vi "Get Connection to Detector.vi"(6 "BAUD":u16, 7 "Mode":enum16{"RTU", "ASCII"}(ring), 8 "error in (no error)":errorcluster, 9 "Порт":u16, 10 "find list":string[](array[string]), 11 "Адрес датчика":u16) -> (0 "error out":errorcluster, 1 "SN":u16, 2 "FW":u16, 3 "VISA Refnum out":refnum<visa-resource-name>, 4 "p_atm":sgl, 5 "Cluster":T1)   [LabVIEW 2020]
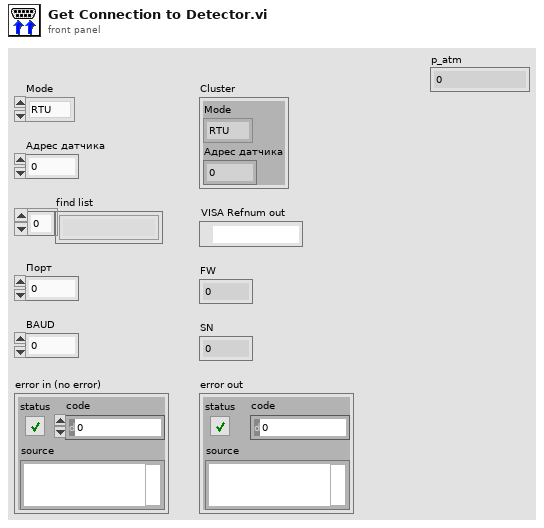
[diagram p1: front panel]
types:
  T1 = cluster{"Mode":enum16{"RTU", "ASCII"}, "Адрес датчика":u16}
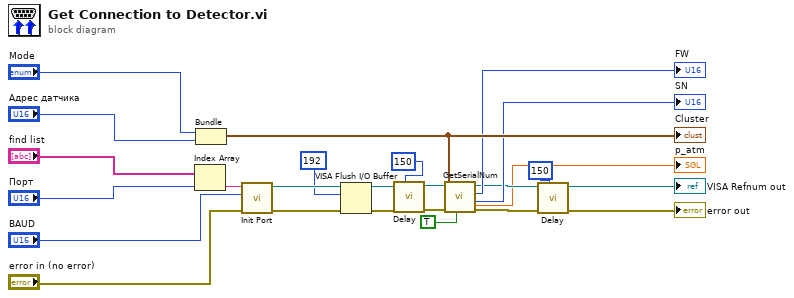
[diagram p0: block diagram]
diagram:
  n1 = Index Array(array="find list", index="Порт") -> (element=w12:string)
  n2 = Bundle("Mode"="Mode", "Адрес датчика"="Адрес датчика") -> (w9:T1)  [unwired: 1 in]
  "Cluster" <- w9
  n3 = call "Init Port.vi"("error in (no error)"="error in (no error)", "BAUD"="BAUD", "String"=w12) -> ("error out"=w24:errorcluster, "VISA Refnum out"=w18:refnum<visa-resource-name>)  [unwired: 7 in]
  n4 = VISA Flush I/O Buffer(VISA resource name=w18, mask (16)=u16 192, error in (no error)=w24) -> (VISA resource name out=w8:refnum<visa-resource-name>, error out=w19:errorcluster)
  n5 = call "Delay.vi"("milliseconds to wait"=u32 150, "error in (no error)"=w19, "VISA Refnum  In"=w8) -> ("error out"=w25:errorcluster, "VISA Refnum out"=w7:refnum<visa-resource-name>)  [unwired: 7 in]
  n6 = call "GetSerialNum.vi"("Enable"=TRUE, "error in (no error)"=w25, "Cluster"=w9, "VISA Refnum in"=w7) -> ("error out"=w23:errorcluster, "Serial num"=→"SN":u16, "Firmware"=→"FW":u16, "VISA Refnum OUT"=w4:refnum<visa-resource-name>, "p_atm"=→"p_atm":sgl)  [unwired: 3 in]
  n7 = call "Delay.vi"("milliseconds to wait"=u32 150, "error in (no error)"=w23, "VISA Refnum  In"=w4) -> ("error out"=→"error out":errorcluster, "VISA Refnum out"=→"VISA Refnum out":refnum<visa-resource-name>)  [unwired: 7 in]
